vi "oscope_oldMethod.vi"() -> ()   [LabVIEW 2020]
panel:
  out "Y":dbl[](array[numeric])
  out "error out":errorcluster
  out "Wvfrm Param.":string
  in  "Oscilloscope":refnum<visa-resource-name>="GPIB0::20::INSTR"
  out "Acqr Param.":string
  in  "Start Point":i32=1
  in  "End Point":i32=2500
  in  "# Average":i32(slide) scale=4.0..128.0
  in  "Waveform Width":u8(knob) min=1 max=2 step=1 scale=1.0..2.0
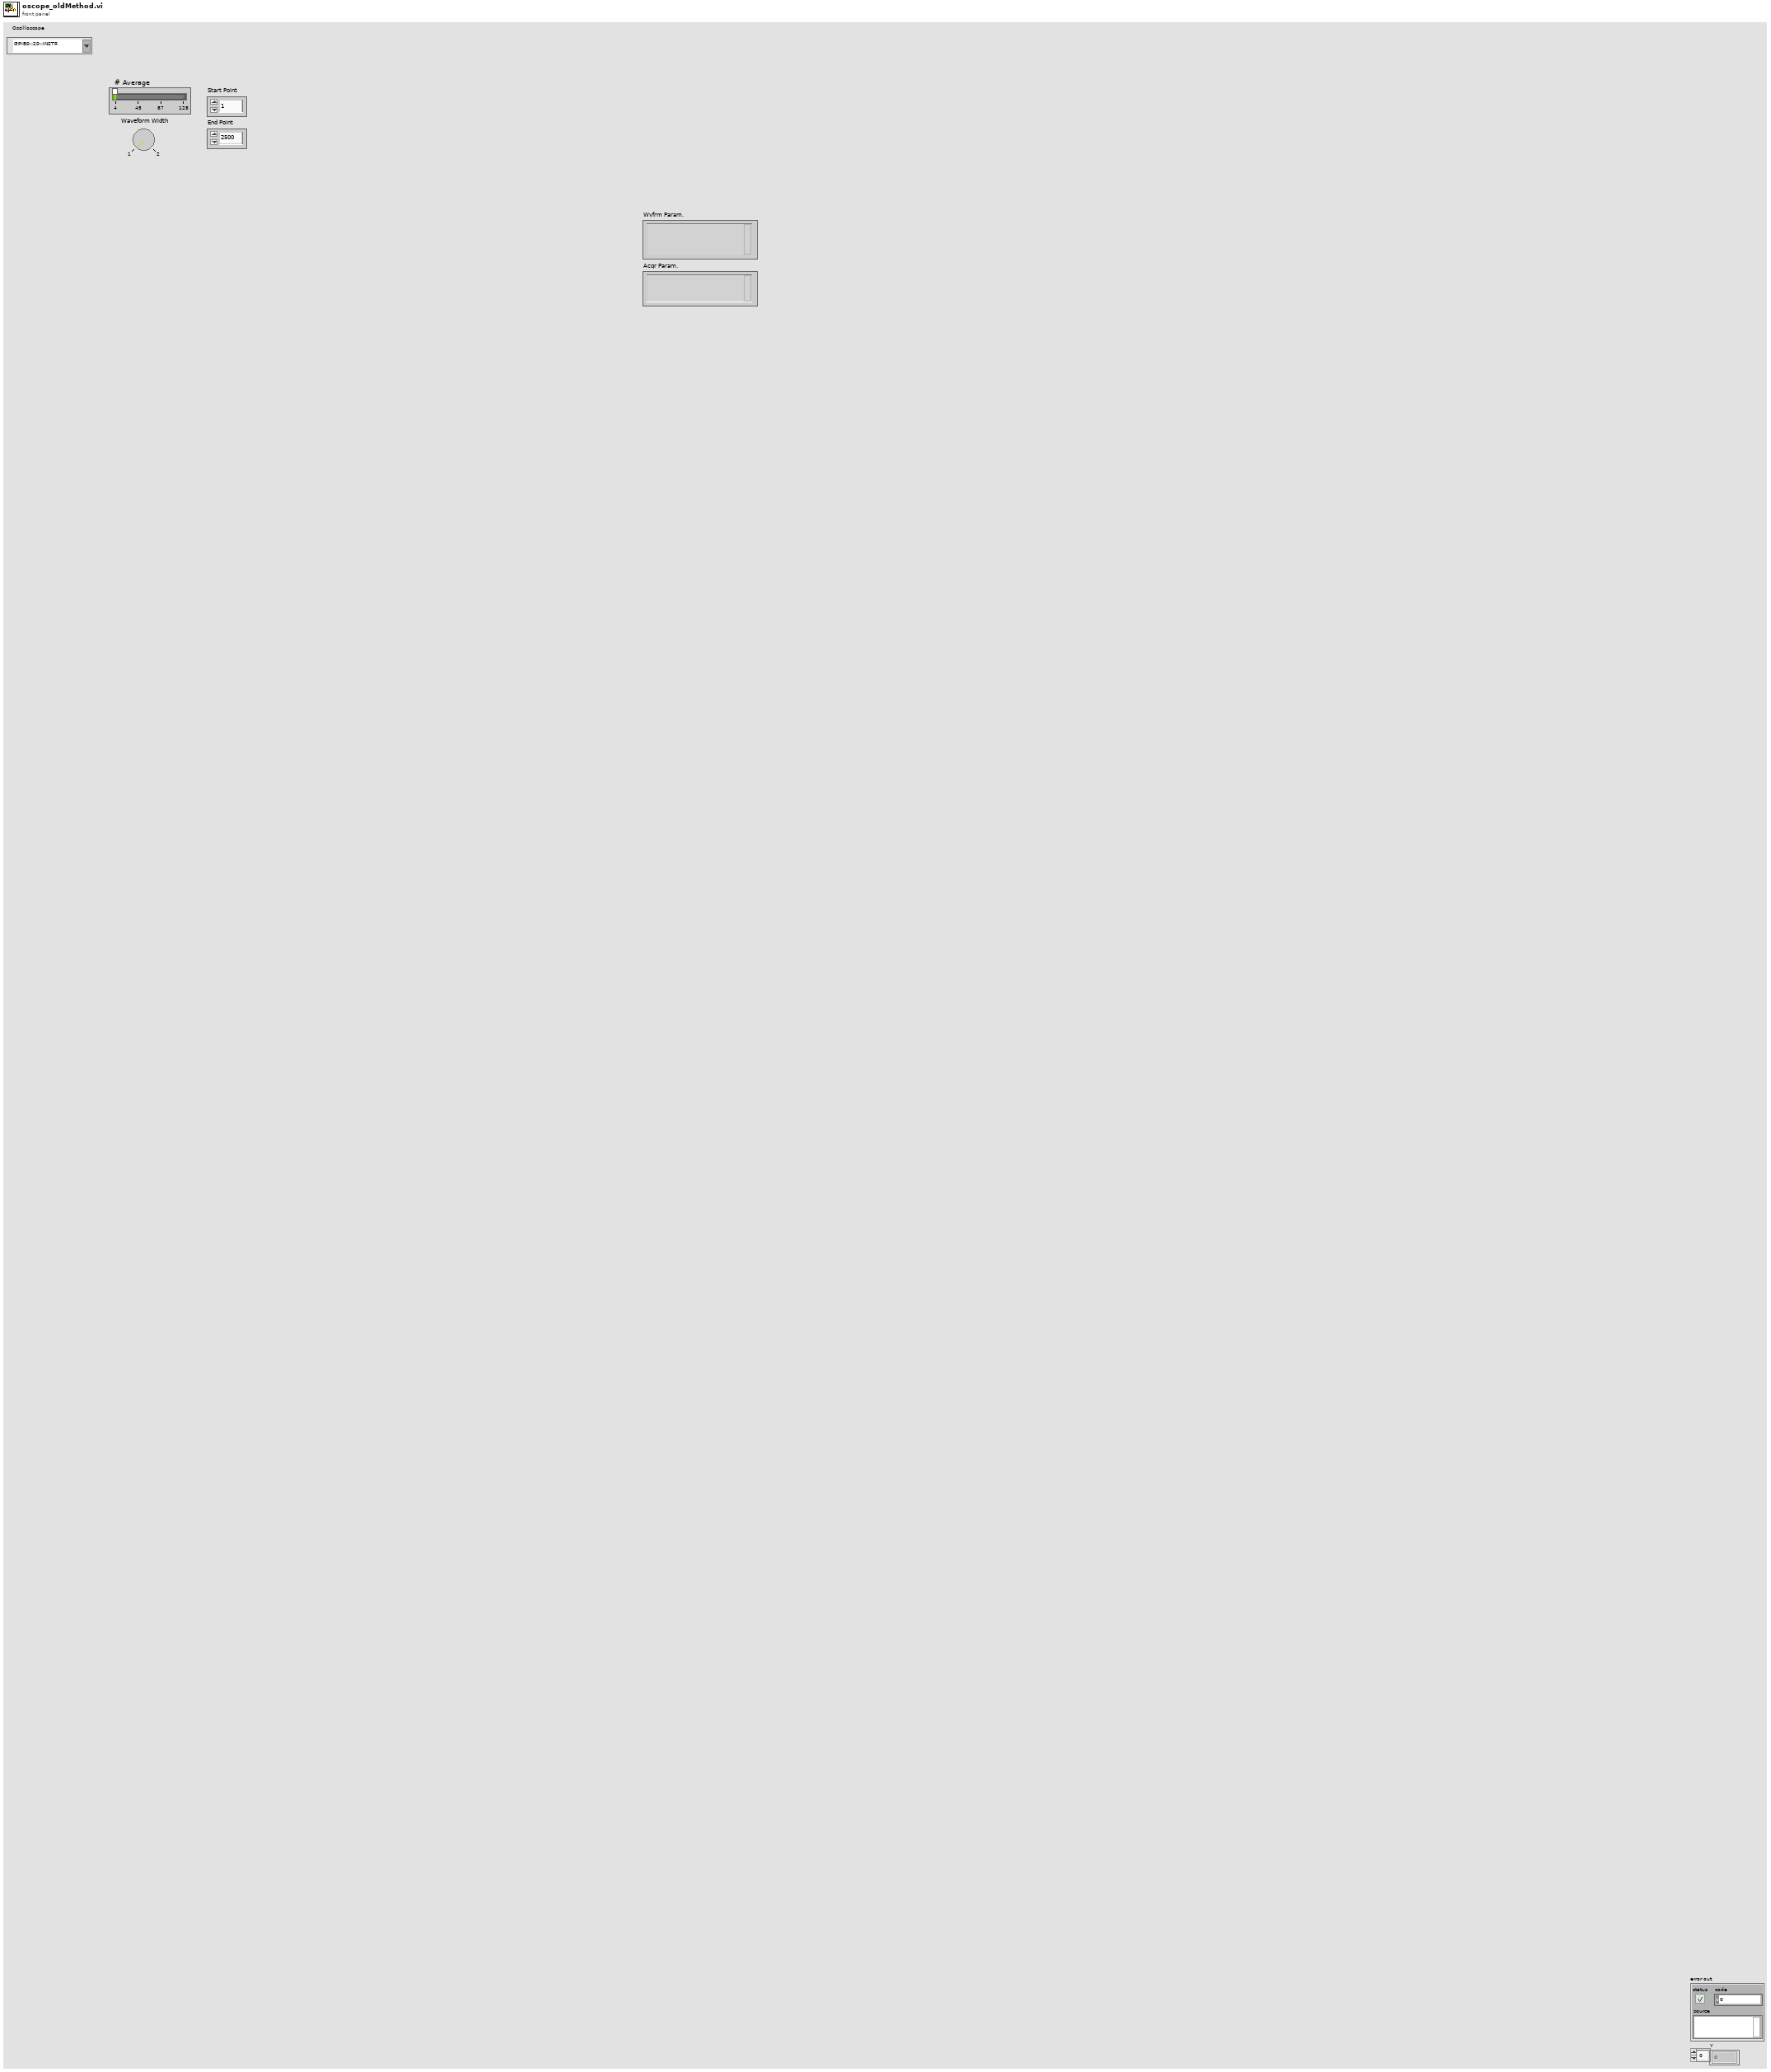
[diagram p1: front panel]
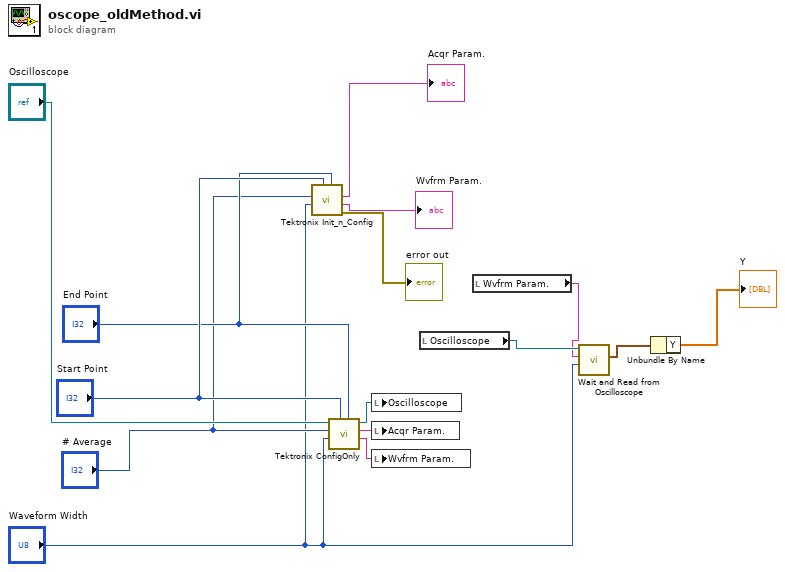
[diagram p0: block diagram]
diagram:
  n1 = call "Tektronix Init_n_Config.vi"("End Point"="End Point", "Start Point"="Start Point", "Waveform Width"="Waveform Width", "# Average"="# Average") -> ("error out"=→"error out":errorcluster, "Waveform Parameters"=→"Wvfrm Param.":string, "Acquire Parameters"=→"Acqr Param.":string)  [unwired: 3 in, 2 out]
  n2 = call "Tektronix ConfigOnly.vi"("End Point"="End Point", "Start Point"="Start Point", "Waveform Width"="Waveform Width", "# Average"="# Average", "Tektronix (0::20:)"="Oscilloscope") -> ("Waveform Parameters"=w14:string, "Acquire Parameters"=w13:string, "VISA resource name out"=w15:refnum<visa-resource-name>)  [unwired: 3 in, 1 out]
  n3 = local write "Oscilloscope"(w15) -> ()
  n4 = local write "Acqr Param."(w13) -> ()
  n5 = local write "Wvfrm Param."(w14) -> ()
  n6 = local read "Oscilloscope"() -> (w5:refnum<visa-resource-name>)
  n7 = local read "Wvfrm Param."() -> (w4:string)
  n8 = call "Wait and Read from Oscilloscope.vi"("Waveform Width"="Waveform Width", "data format"=w4, "VISA resource name"=w5) -> ("output waveform 2"=w2:waveform(dbl))  [unwired: 5 in, 3 out]
  n9 = Unbundle By Name(w2) -> ("Y"=→"Y":dbl[])
